vi "FindDepsChainPath.vi"(9 "Dependency Path":string, 10 "Current Dependency":string, 11 "Dependency Map":map{string, string[]}(c390)) -> (3 "Dependency Chain []":string[](array[string]))   [LabVIEW 2019, in "Hawkeye.lvlib"]
uses:
  Hawkeye.lvlib
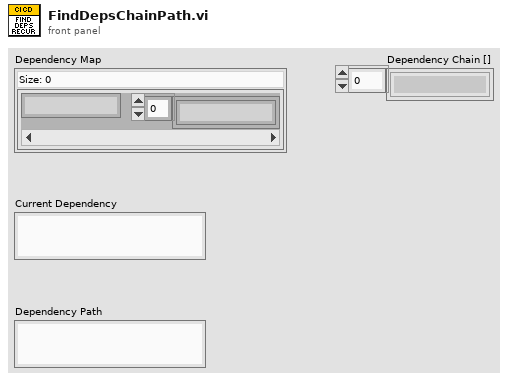
[diagram p1: front panel]
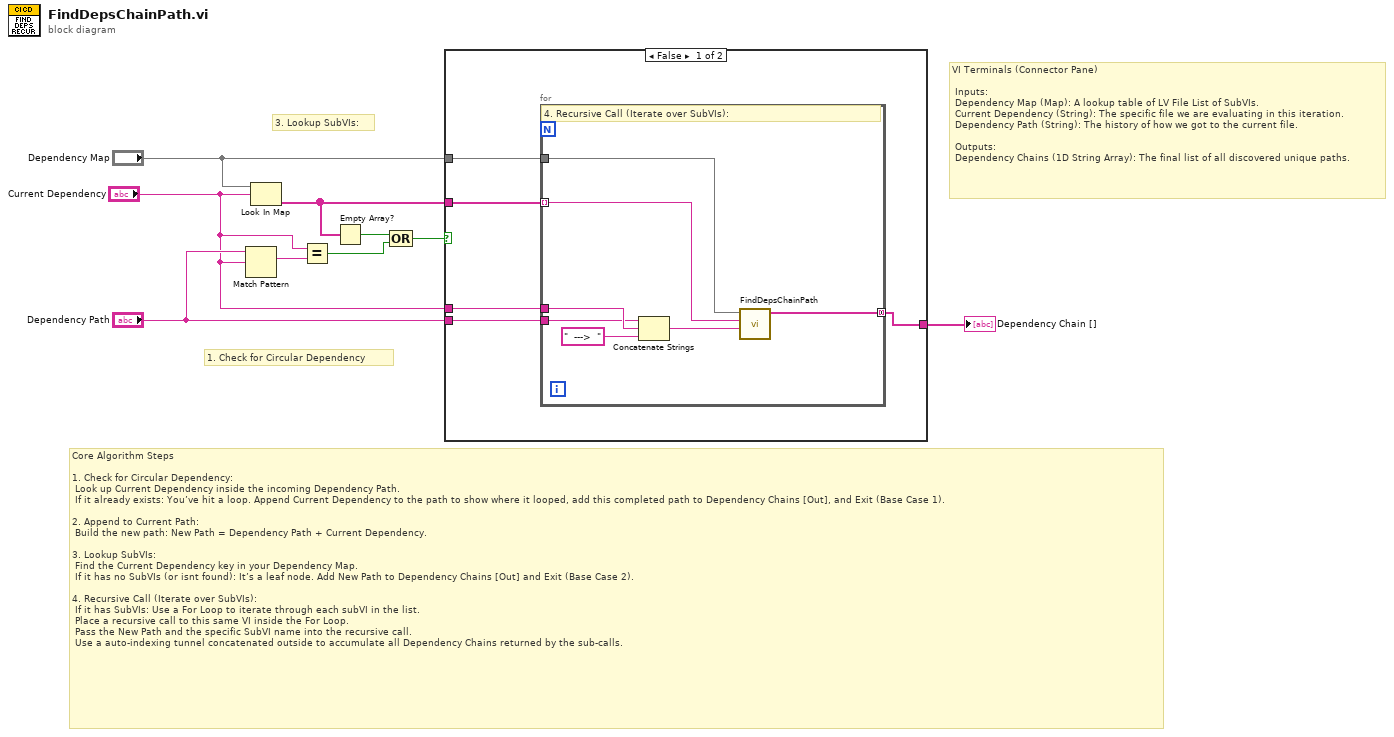
[diagram p0: block diagram]
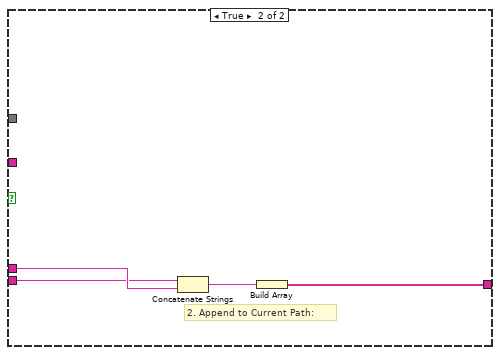
[diagram p2: hidden frame]
diagram:
  # "3. Lookup SubVIs:"
  # "1. Check for Circular Dependency"
  # "Core Algorithm Steps\n\n1. Check for Circular Dependency:\n Look up Current Dependency inside the incoming Dependency Path.\n If it already exists: You’ve hit a loop. Append Current Dependency to the path to show where it looped, add this completed path to Dependency Chains [Out], and Exit (Base Case 1).\n\n2. Append to Current Path:\n Build the new path: New Path = Dependency Path + Current Dependency.\n\n3. Lookup SubVIs:\n Find the Current Dependency key in your Dependency Map.\n If it has no SubVIs (or isnt found): It’s a leaf node. Add New Path to Dependency Chains [Out] and Exit (Base Case 2).\n\n4. Recursive Call (Iterate over SubVIs):\n If it has SubVIs: Use a For Loop to iterate through each subVI in the list.\n Place a recursive call to this same VI inside the For Loop.\n Pass the New Path and the specific SubVI name into the recursive call.\n Use a auto-indexing tunnel concatenated outside to accumulate all Dependency Chains returned by the sub-calls."
  # "VI Terminals (Connector Pane)\n\n Inputs:\n Dependency Map (Map): A lookup table of LV File List of SubVIs.\n Current Dependency (String): The specific file we are evaluating in this iteration.\n Dependency Path (String): The history of how we got to the current file.\n\n Outputs:\n Dependency Chains (1D String Array): The final list of all discovered unique paths."
  n1 = Match Pattern(string="Dependency Path", regular expression="Current Dependency") -> (match substring=w2:string)  [unwired: 1 in, 3 out]
  n2 = Look In Map(map="Dependency Map", key="Current Dependency") -> (value=w7:string[])  [unwired: 1 in, 1 out]
  n3 = Equal?(x="Current Dependency", y=w2) -> (x = y?=w3:bool)
  n4 = Empty Array?(array=w7) -> (empty?=w9:bool)
  n5 = Compound Arithmetic op=OR(w9, w3) -> (w4:bool)
  n6 = case shown="False" w4 {
    tunnel: "Dependency Map" -> [w14 _]
    tunnel: w7 -> [w13 _]
    tunnel: "Current Dependency" -> [w12 w25]
    tunnel: "Dependency Path" -> [w11 w22]
    tunnel: [w10 w23] -> w8
    frame False {
      n7 = for {
        tunnel: w14 -> [w21]
        tunnel: w13 -> [w20] mode=indexing
        tunnel: w12 -> [w19]
        tunnel: w11 -> [w17]
        tunnel: [w16] -> w10 mode=concatenating
        # "4. Recursive Call (Iterate over SubVIs):"
        n8 = Concatenate Strings(w17, w19, "  --->  " ("string")) -> (w18:string)
        n9 = call "FindDepsChainPath.vi"("Dependency Path"=w18, "Current Dependency"=w20, "Dependency Map"=w21) -> ("Dependency Chain []"=w16:string[])  [unwired: 8 in]
      }
    }
    frame True {
      # "2. Append to Current Path:"
      n10 = Concatenate Strings(w22, w25) -> (w24:string)
      n11 = Build Array(w24) -> (w23:string[])
    }
  }
  "Dependency Chain []" <- w8
